vi "ad single.vi"(7 "databuf":sgl, 8 "error in (no error)":errorcluster caption="错误输入（无错误）", 9 "ad_range":i32, 10 "ad_os":i32, 11 "dev":i32) -> (0 "error out":errorcluster caption="错误输出", 3 "function return":i32, 5 "databuf out":sgl)   [LabVIEW 2018, in "恒凯采集卡.lvlib"]
doc: "int ad_single(int dev,int ad_os,int ad_range,float* databuf);"
uses:
  data/Usb_Daq_V52_32.dll
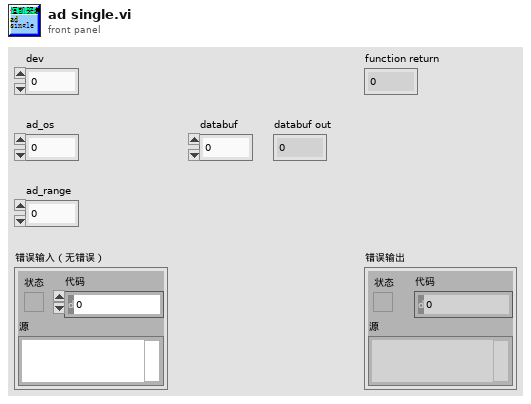
[diagram p1: front panel]
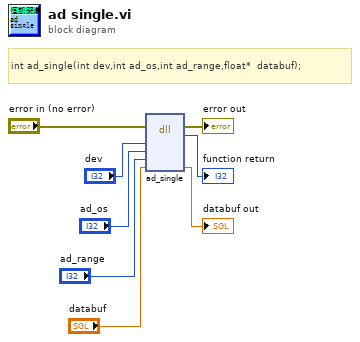
[diagram p0: block diagram]
diagram:
  # "int ad_single(int dev,int ad_os,int ad_range,float*  databuf);"
  n1 = dll-call lib="D:/ProgramFiles/NI/LabVIEW 2018/user.lib/Usb_Daq_V52_32/Usb_Daq_V52_32.*" fn="ad_single"(error in="error in (no error)", "dev"="dev", "ad_os"="ad_os", "ad_range"="ad_range", "databuf"="databuf") -> (error out=→"error out":errorcluster, →"function return":i32, "databuf"=→"databuf out":sgl)  [unwired: 5 in, 1 out]
